vi "StartRCMWithParameters_RCM.vi"(0 "Display State In":T1={"RCM File Path"=path "", "Left"=300, "Top"=300, "Font Name"="Tahoma", "Font Size"=13, "Font Color"=0, "Separator Color"=9868950, "Frame Color"=9868950, "Overlay Color"=26367}, 1 "VI Refnum":refnum<vi>, 5 "RCM File Path":path, 7 "Position":cluster{"left":u32, "top":u32}, 9 "Container State":T2, 11 "error in (no error)":errorcluster) -> (4 "Display State Out":T1={"RCM File Path"=path "", "Left"=300, "Top"=300, "Font Name"="Tahoma", "Font Size"=13, "Font Color"=0, "Separator Color"=9868950, "Frame Color"=9868950, "Overlay Color"=26367}, 15 "error out":errorcluster)   [LabVIEW 2009, in "RCM.xctl"]
uses:
  RCM.xctl
  <vilib>/_xctls/Container State.ctl
  Ability/State_RCM.ctl
  <vilib>/_xctls/XControlSupport.lvlib
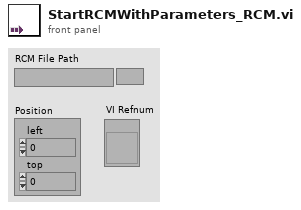
[diagram p1: front panel]
types:
  T1 = typedef "RCM.xctl/State_RCM.ctl" = cluster{"RCM File Path":path, "Left":u32, "Top":u32, "Font Name":string, "Font Size":i16, "Font Color":u32, "Separator Color":u32, "Frame Color":u32, "Overlay Color":u32}
  T2 = typedef "XControlSupport.lvlib/Container State.ctl" = cluster{"Indicator?":bool, "Run Mode?":bool, " Refnum":refnum<vi>}
  T3 = cluster{"position":cluster{"left":u32, "top":u32}, "font":cluster{"name":string, "size":i16, "color":u32}, "seperator color":u32, "frame color":u32, "overlay color":u32}
  T4 = typedef "LVRectTypeDef.ctl" = cluster{"left":i16, "top":i16, "right":i16, "bottom":i16}
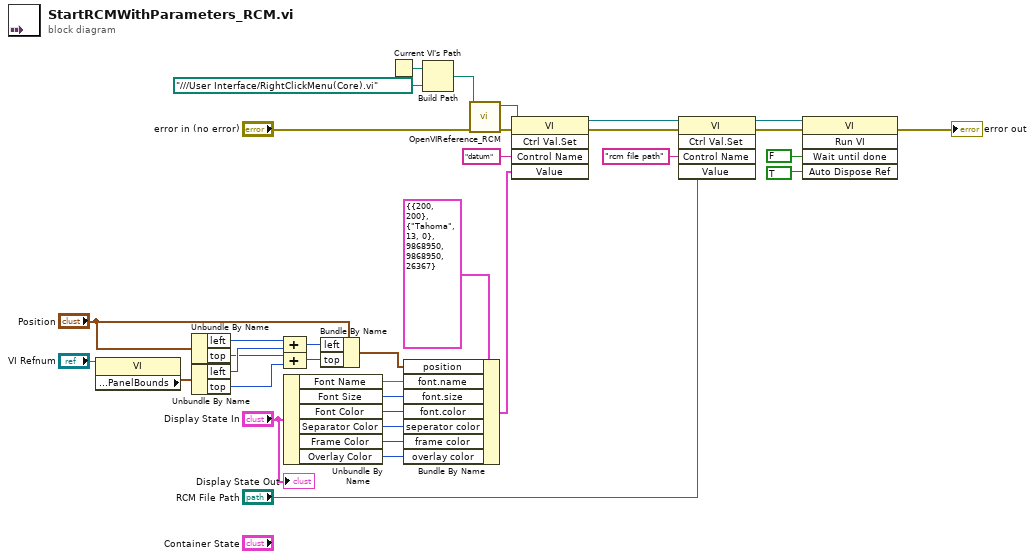
[diagram p0: block diagram]
diagram:
  n1 = property class="VI"(reference="VI Refnum") -> ("Front Panel.PanelBounds"=w8:T4)  [unwired: 1 in, 2 out]
  n2 = Unbundle By Name("Position") -> ("left"=w4:u32, "top"=w1:u32)
  n3 = Unbundle By Name(w8) -> ("left"=w2:i16, "top"=w3:i16)
  n4 = Compound Arithmetic op=ADD(w4, w2) -> (w6:u32)
  n5 = Compound Arithmetic op=ADD(w1, w3) -> (w5:u32)
  n6 = Unbundle By Name("Display State In") -> ("Font Name"=w33:string, "Font Size"=w32:i16, "Font Color"=w31:u32, "Separator Color"=w30:u32, "Frame Color"=w29:u32, "Overlay Color"=w28:u32)
  n7 = Bundle By Name(cluster="Position", "left"=w6, "top"=w5) -> (w10:cluster{"left":u32, "top":u32})
  n8 = Current VI's Path() -> (path=w17:path)
  n9 = Bundle By Name(cluster=T3 {"position"={"left"=200, "top"=200}, "font"={"name"="Tahoma", "size"=13, "color"=0}, "seperator color"=9868950, "frame color"=9868950, "overlay color"=26367} ("datum"), "position"=w10, "font.name"=w33, "font.size"=w32, "font.color"=w31, "seperator color"=w30, "frame color"=w29, "overlay color"=w28) -> (w20:T3)
  n10 = Build Path(base path=w17, name or relative path=path "../../../User Interface/RightClickMenu(Core).vi" ("vi path")) -> (appended path=w11:path)
  n11 = call "OpenVIReference_RCM.vi"("error in (no error)"="error in (no error)", "path"=w11) -> ("error out"=w14:errorcluster, "vi reference"=w12:refnum<vi>)  [unwired: 8 in]
  n12 = invoke class="VI" method="Ctrl Val.Set"(reference=w12, error in=w14, "Control Name"="datum", "Value"=w20) -> (reference out=w21:refnum<vi>, error out=w22:errorcluster)  [unwired: 1 in, 3 out]
  n13 = invoke class="VI" method="Ctrl Val.Set"(reference=w21, error in=w22, "Control Name"="rcm file path", "Value"="RCM File Path") -> (reference out=w24:refnum<vi>, error out=w23:errorcluster)  [unwired: 1 in, 3 out]
  n14 = invoke class="VI" method="Run VI"(reference=w24, error in=w23, "Wait until done"=FALSE ("Wait Until Done"), "Auto Dispose Ref"=TRUE ("Auto Dispose Reference")) -> (error out=→"error out":errorcluster)  [unwired: 1 in, 4 out]
  "Display State Out" <- "Display State In"
